vi "Apply View to All Controls.vi"(7 "View Mode":T3, 8 "error in (no error)":errorcluster, 11 "Application Data in":T1) -> (0 "error out":errorcluster, 3 "Application Data out":T1)   [LabVIEW 2017]
uses:
  View Mode.ctl
  Application Data.ctl
  DSF Configuration API/1.0.0/Public/Controls/DSF Config Data RefNum.ctl
  Window State.ctl
  DSF Configuration API/1.0.0/DSF Configuration API.lvlib
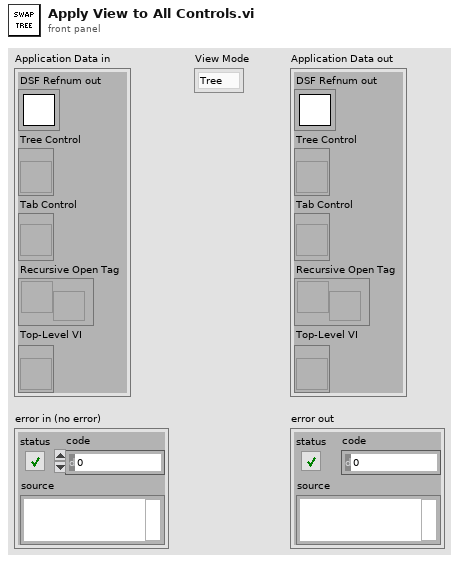
[diagram p1: front panel]
types:
  T1 = typedef "Application Data.ctl" = cluster{"DSF Refnum out":T2, "Tree Control":refnum<vi>, "Tab Control":refnum<vi>, "Recursive Open Tag":refnum<user-event>, "Top-Level VI":refnum<vi>}
  T2 = typedef "DSF Configuration API.lvlib/DSF Config Data RefNum.ctl" = refnum<k1>
  T3 = typedef "View Mode.ctl" = enum16{"Tree", "List"}
  T4 = typedef "Window State.ctl" = enum32{"Blank", "Loading", "No File Loaded", "Plugin", "Group", "Transfer", "Channel", "Settings"}
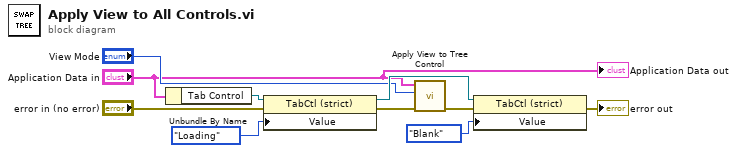
[diagram p0: block diagram]
diagram:
  n1 = Unbundle By Name("Application Data in") -> ("Tab Control"=w4:refnum<vi>)
  n2 = property class="TabCtl (strict)"(reference=w4, error in="error in (no error)", "Value"=Window_State."Loading") -> (reference out=w3:refnum<vi>, error out=w9:errorcluster)
  n3 = call "Apply View to Tree Control.vi"("error in (no error)"=w9, "View Mode"="View Mode", "Application Data"="Application Data in") -> ("error out"=w5:errorcluster)  [unwired: 8 in]
  n4 = property class="TabCtl (strict)"(reference=w3, error in=w5, "Value"=Window_State."Blank") -> (error out=→"error out":errorcluster)  [unwired: 1 out]
  "Application Data out" <- "Application Data in"
